vi "Tester.vi"() -> ()   [LabVIEW 2026]
uses:
  fissionReactor_State.ctl
  Fission Reactor Build Properties.ctl
  Fission Reactor Build Specifications.ctl
panel:
  out "JSON":string
  in  "State":T1={"Burn Rate"=0.0, "Formed"=FALSE, "Reactor Build Properties"={"Fuel Rods"=0, "Control Rods"=0, "Volume (m³)"=0, "Fuel Surface Area (m²)"=0, "Cooled Coolant Tank (mB)"=0, "Fuel Capacity (mB)"=0, "Heat Capacity (J/K)"=0.0, "Max Burn Rate"=0, "Max Heating Rate (mB/t)"=0, "Boil Efficiency"=0.0, "Coolant Type"=enum."Water", "Heated Coolant Tank (mB)"=0}, "Fission Reactor Build Specifications"={"Length (m)"=3, "Width (m)"=3, "Height (m)"=4, "Coolant Type"=enum."Water"}} {"Fission Reactor Build Specifications"."Height (m)" min=4 max=18 step=1; "Fission Reactor Build Specifications"."Width (m)" min=3 max=18 step=1; "Fission Reactor Build Specifications"."Length (m)" min=3 max=18 step=1; "Reactor Build Properties"."Boil Efficiency" format="%#.6g"}
  in  "Function":string
  in  "Mode":enum16{"Publish", "Read", "Handle", "Command"}(ring)
  in  "Peripheral":string
  in  "stop":bool
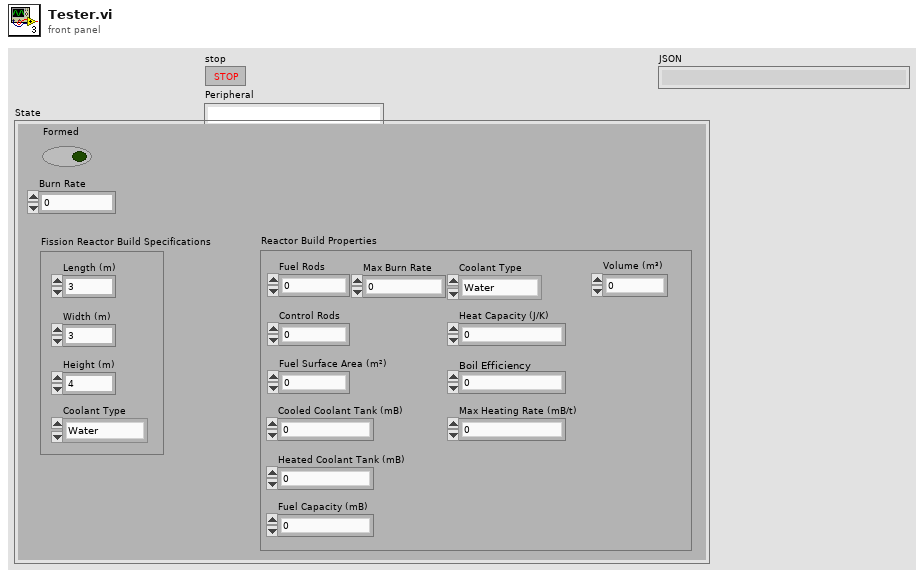
[diagram p1: front panel]
types:
  T1 = typedef "fissionReactor_State.ctl" = cluster{"Burn Rate":dbl, "Formed":bool, "Reactor Build Properties":T2, "Fission Reactor Build Specifications":T3}
  T2 = typedef "Fission Reactor Build Properties.ctl" = cluster{"Fuel Rods":i32, "Control Rods":i32, "Volume (m³)":i32, "Fuel Surface Area (m²)":i32, "Cooled Coolant Tank (mB)":i32, "Fuel Capacity (mB)":i64, "Heat Capacity (J/K)":dbl, "Max Burn Rate":i64, "Max Heating Rate (mB/t)":i64, "Boil Efficiency":dbl, "Coolant Type":enum16{"Water", "Sodium"}, "Heated Coolant Tank (mB)":i64}
  T3 = typedef "Fission Reactor Build Specifications.ctl" = cluster{"Length (m)":i32, "Width (m)":i32, "Height (m)":i32, "Coolant Type":enum16{"Water", "Sodium"}}
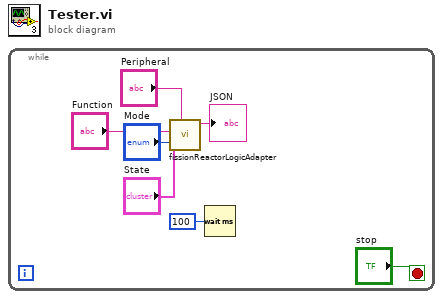
[diagram p0: block diagram]
diagram:
  n1 = while {
    stop <- "stop" stop-if-true
    n2 = call "fissionReactorLogicAdapter.vi"("Peripheral"="Peripheral", "State"="State", "Function"="Function", "Mode"="Mode") -> ("JSON"=→"JSON":string)  [unwired: 7 in]
    n3 = Wait (ms)(milliseconds to wait=u32 100) -> ()  [unwired: 1 out]
  }
